vi "LibXML_CheckElementExists.vi"(8 "error in":errorcluster, 9 "queryString":string, 10 "rootnode (root of doc)":u32, 11 "doc":u32) -> (0 "error out":errorcluster, 2 "exists":bool, 3 "doc copy out":u32)   [LabVIEW 2019, in "Tools.lvlib" / "LibXML.lvlib"]
doc: "This VI searches the XMLDocument with the querystring according to the XPATH protocol and returns the number (length) of the nodes found as well as the first Node found. If not found \"not found\"will be set true"
uses:
  LibXML.lvlib
  Error Cluster From Error Code_subroutine.vi
  <vilib>/Utility/error.llb/Trim Whitespace.vi
panel:
  # "This software is FREE licensed under the GNU Lesser General Public License"
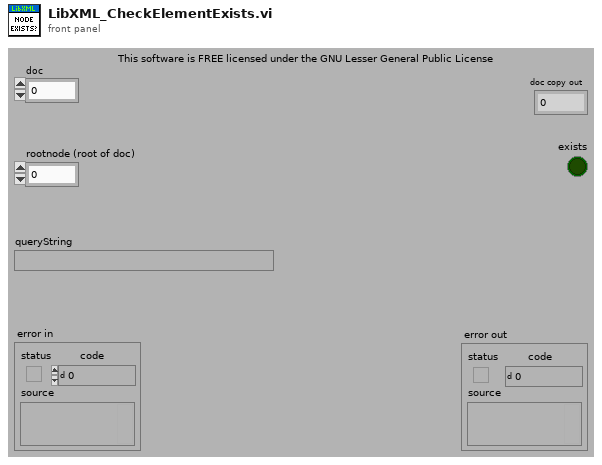
[diagram p1: front panel]
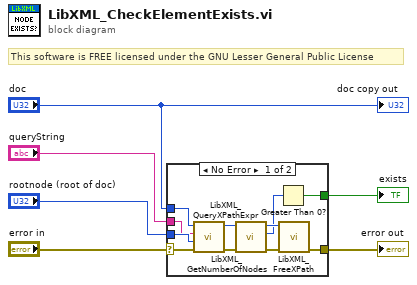
[diagram p0: block diagram]
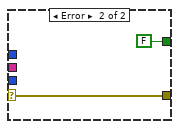
[diagram p2: hidden frame]
diagram:
  # "This software is FREE licensed under the GNU Lesser General Public License"
  n1 = case shown="No Error" "error in" {
    selector: "error in" -> [w17 w19]
    tunnel: [w14 w19] -> w6
    tunnel: "doc" -> [w16 _]
    tunnel: [w15 FALSE ("Not found")] -> w4
    tunnel: "rootnode (root of doc)" -> [w8 _]
    tunnel: "queryString" -> [w7 _]
    frame No Error {
      n2 = call "LibXML_QueryXPathExpr.vi"("error in"=w17, "rootnode (root of doc)"=w8, "XPathExpr"=w7, "doc"=w16) -> ("error out"=w13:errorcluster, "xmlXPathObj"=w11:u32)  [unwired: 6 in]
      n3 = call "LibXML_GetNumberOfNodes.vi"("error in (no error)"=w13, "XPathObj"=w11) -> ("error out"=w12:errorcluster, "#ofNodes"=w9:i32, "XPathObj out"=w10:u32)  [unwired: 7 in]
      n4 = Greater Than 0?(x=w9) -> (x > 0?=w15:bool)
      n5 = call "LibXML_FreeXPath.vi"("error in"=w12, "XPathObj"=w10) -> ("error out"=w14:errorcluster)  [unwired: 9 in]
    }
    frame Error {
    }
  }
  "error out" <- w6
  "exists" <- w4
  "doc copy out" <- "doc"
